vi "Routing Channel Page.vi"(8 "error in (no error)":errorcluster, 11 "Node Ptr":T8 format="%.0x") -> (0 "error out":errorcluster)   [LabVIEW 2017, in "Routing and Faulting System Explorer.lvlib"]
uses:
  Routing and Faulting System Explorer.lvlib
  <vilib>/NI Veristand/Custom Device API/Custom Device Item Ref.ctl
  State-Value Row.ctl
  Connection Row.ctl
  State Control.ctl
  Shared/UI Common/Duplicate Button.ctl
  Shared/UI Common/Add Button.ctl
  Shared/UI Common/Remove Button.ctl
  Routing Channel Page Controls.ctl
  2402a215-ce2b-4427-ab28-3f6d8102afb6.vi
  Shared/UI Common/Set Control Value.vi
  <vilib>/NI VeriStand/Custom Device API/Custom Device API.lvlib
  Scripting/Routing and Faulting Scripting.lvlib
  Shared/UI Common/UI Common.lvlib
panel:
  in  "Configuration Tab":T1(tab)
  in  "show module":bool
  in  "Connections":T2[](array[typedef])
  in  "State Value":string
  in  "State Description":string
  in  "Add Connection":T3
  in  "State Name":T4
  in  "Duplicate State":T5
  in  "Remove State":T6
  in  "Add State":T3
  out "States":T7[](array[typedef])
  in  "Initial State":string(combo)
  in  "Routing Channel Name":string
  in  "SHDocVw.IWebBrowser":refnum<k7>(container)
  in  "Description":string
  # "Source"
  # "Destination"
  # "State Name"
  # "State Value"
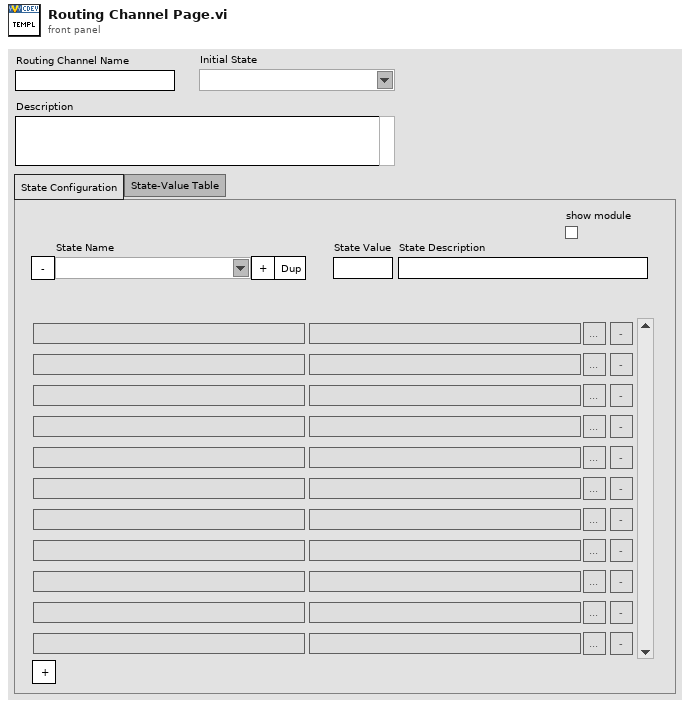
[diagram p1: front panel]
types:
  T1 = enum32{"State Configuration", "State-Value Table"}
  T2 = typedef "Routing and Faulting System Explorer.lvlib/Connection Row.ctl" = cluster{"Source":string, "Destination":string, "Edit":bool, "Remove":bool}
  T3 = typedef "UI Common.lvlib/Add Button.ctl" = bool
  T4 = typedef "Routing and Faulting System Explorer.lvlib/State Control.ctl" = string
  T5 = typedef "UI Common.lvlib/Duplicate Button.ctl" = bool
  T6 = typedef "UI Common.lvlib/Remove Button.ctl" = bool
  T7 = typedef "Routing and Faulting System Explorer.lvlib/State-Value Row.ctl" = cluster{"State":string, "State Value":string}
  T8 = typedef "Custom Device API.lvlib/Custom Device Item Ref.ctl" = u64
  T9 = typedef "Routing and Faulting System Explorer.lvlib/Routing Channel Page Controls.ctl" = cluster{"Description":refnum<vi>, "Routing Channel Name":refnum<vi>, "Initial State":refnum<vi>, "Configuration Tab":refnum<vi>, "States":refnum<vi>, "State Value":refnum<vi>, "State Name":refnum<vi>, "State Description":refnum<vi>, "Connections":refnum<vi>}
  T10 = typedef "Routing and Faulting System Explorer.lvlib/Channel Editor State.ctl" = cluster{"Controller":string, "Possible Connections":cluster{"Module":string, "Possible Connections":T11[]}[], "Alias Mappings UI":T12[], "Mappings by Module UI":T13[]}
  T11 = typedef "Routing and Faulting Hardware API.lvlib/Possible Connections for Endpoint.ctl" = cluster{"Source":string, "Destinations":string[]}
  T12 = typedef "Routing and Faulting Shared.lvlib/Alias Mapping.ctl" = cluster{"Endpoint":string, "Alias":string}
  T13 = typedef "Routing and Faulting System Explorer.lvlib/Alias Map by Module.ctl" = cluster{"Module":string, "Alias Map":cluster{"Aliases":string[], "Endpoints":string[]}}
  T14 = typedef "Custom Device API.lvlib/Custom Device Commands.ctl" = enum16{"Default", "Item renamed", "Shutdown", "Dynamic button pressed"}
  T15 = typedef "Routing and Faulting Shared.lvlib/Connection.ctl" = cluster{"Module":string, "Source":string, "Destination":string}
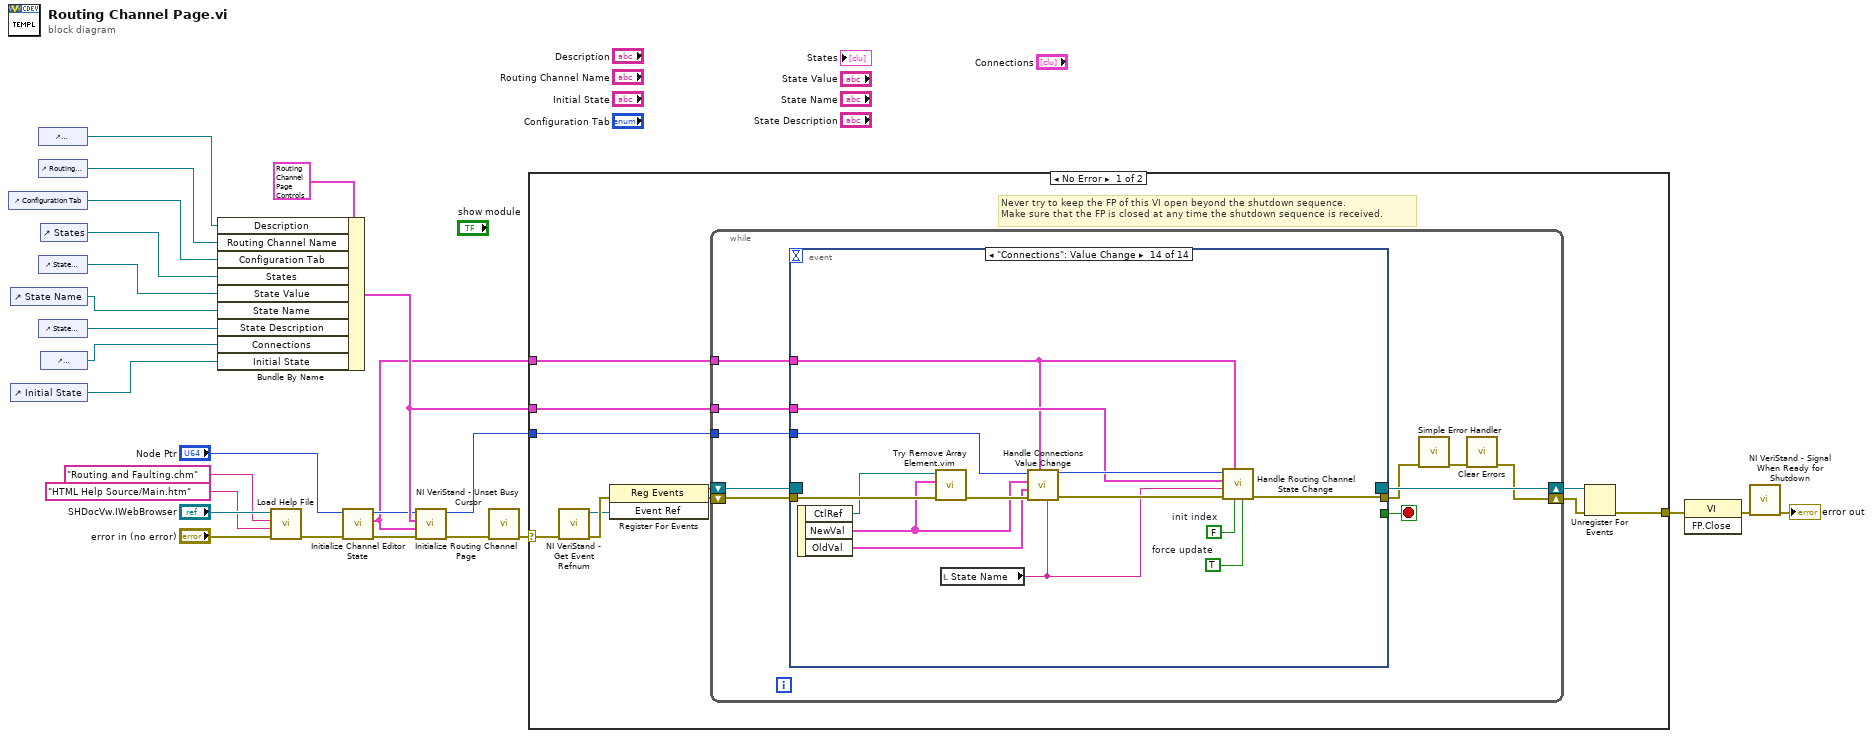
[diagram p0: block diagram]
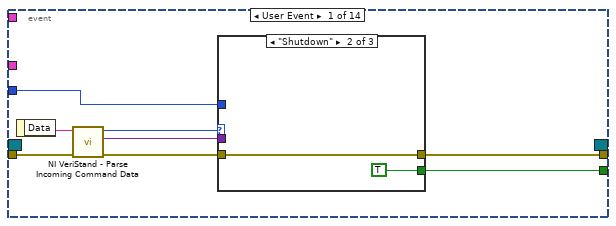
[diagram p2: hidden frame]
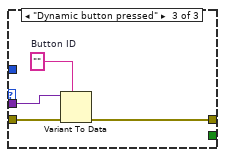
[diagram p4: hidden frame]
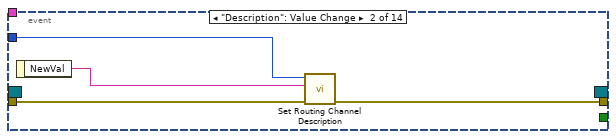
[diagram p5: hidden frame]
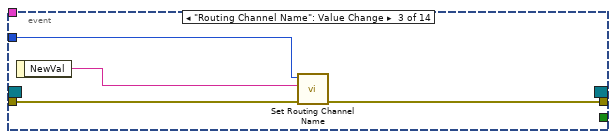
[diagram p6: hidden frame]
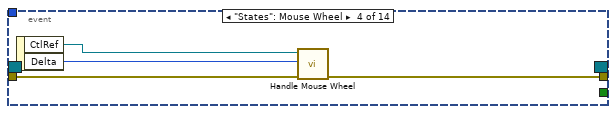
[diagram p7: hidden frame]
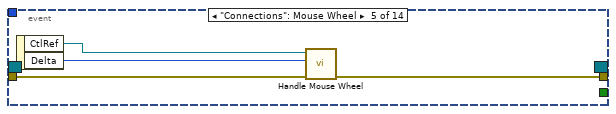
[diagram p8: hidden frame]
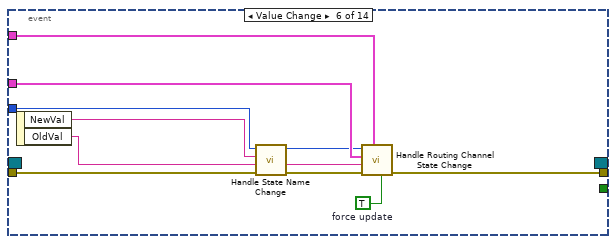
[diagram p9: hidden frame]
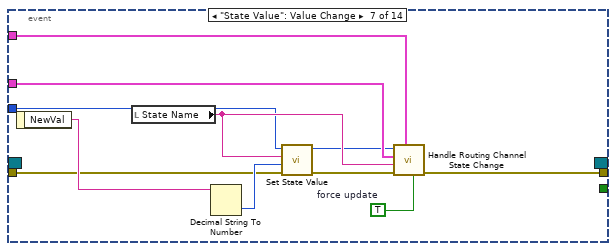
[diagram p10: hidden frame]
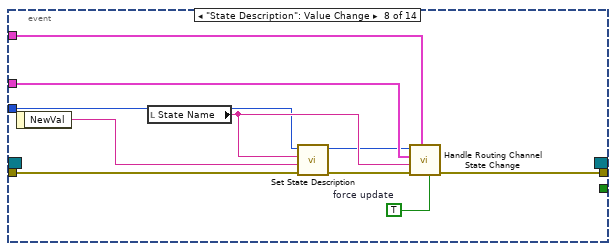
[diagram p11: hidden frame]
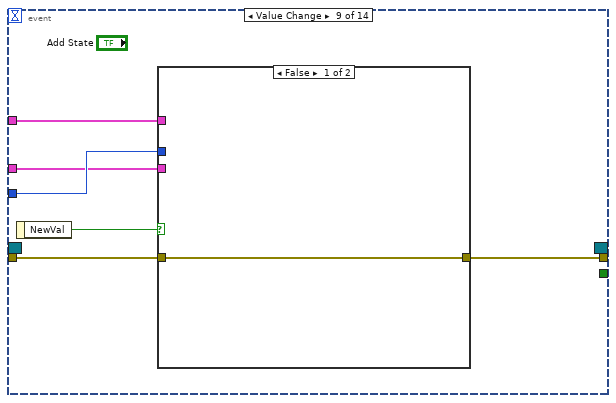
[diagram p12: hidden frame]
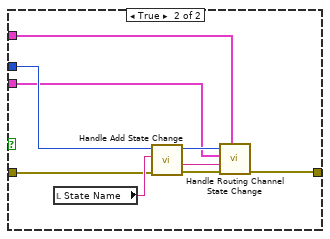
[diagram p13: hidden frame]
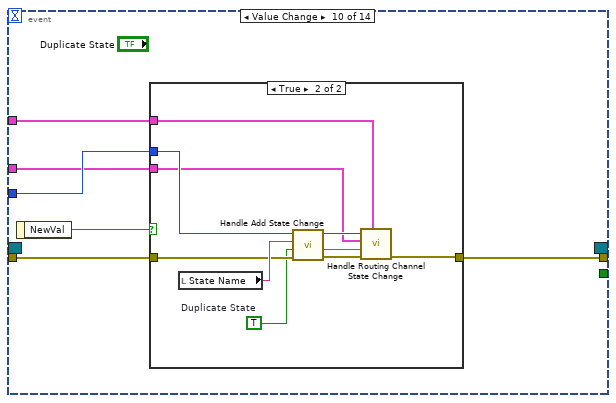
[diagram p14: hidden frame]
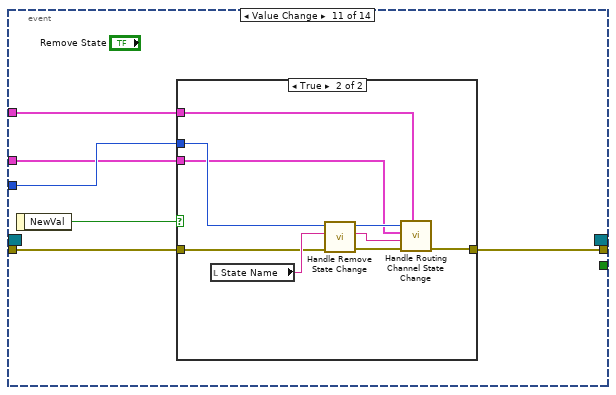
[diagram p16: hidden frame]
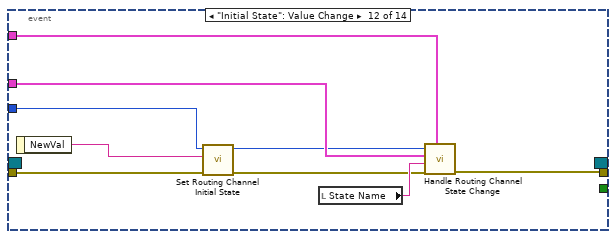
[diagram p18: hidden frame]
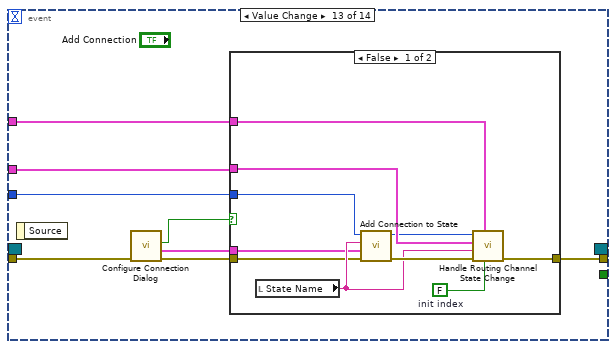
[diagram p19: hidden frame]
diagram:
  n1 = control-ref of="Configuration Tab"() -> (w21:refnum<vi>)
  n2 = control-ref of="State Name"() -> (w12:refnum<vi>)
  n3 = control-ref of="Initial State"() -> (w8:refnum<vi>)
  n4 = control-ref of="Description"() -> (w22:refnum<vi>)
  n5 = control-ref of="Routing Channel Name"() -> (w6:refnum<vi>)
  n6 = control-ref of="State Value"() -> (w19:refnum<vi>)
  n7 = control-ref of="State Description"() -> (w7:refnum<vi>)
  n8 = control-ref of="States"() -> (w20:refnum<vi>)
  n9 = control-ref of="Connections"() -> (w13:refnum<vi>)
  n10 = Bundle By Name(cluster=T9 {"Description"=refnum, "Routing Channel Name"=refnum, "Initial State"=refnum, "Configuration Tab"=refnum, "States"=refnum, "State Value"=refnum, "State Name"=refnum, "State Description"=refnum, "Connections"=refnum} ("Routing Channel Page Controls"), "Description"=w22, "Routing Channel Name"=w6, "Configuration Tab"=w21, "States"=w20, "State Value"=w19, "State Name"=w12, "State Description"=w7, "Connections"=w13, "Initial State"=w8) -> (w9:T9)
  n11 = call "Load Help File.vi"("error in (no error)"="error in (no error)", "HTML File to Load"="HTML Help Source/Main.htm" ("HTML File"), "Main CHM File"="Routing and Faulting.chm" ("CD_CHM_FileName"), "Browser"="SHDocVw.IWebBrowser") -> ("error out"=w4:errorcluster)  [unwired: 7 in]
  n12 = call "Initialize Channel Editor State.vi"("error in (no error)"=w4, "Routing Channel Ref in"="Node Ptr") -> ("error out"=w2:errorcluster, "Channel Editor State"=w1:T10, "Routing Channel Ref out"=w3:T8)  [unwired: 7 in]
  n13 = call "Initialize Routing Channel Page.vi"("error in (no error)"=w2, "Channel Editor State"=w1, "Routing Channel Page Controls"=w9, "Routing Channel Ref in"=w3) -> ("error out"=w10:errorcluster, "Routing Channel Ref out"=w11:T8)  [unwired: 6 in]
  n14 = call <vilib>:"NI VeriStand - Unset Busy Cursor.vi"("error in (no error)"=w10) -> ("error out"=w23:errorcluster)  [unwired: 10 out]
  n15 = case shown="No Error" w23 {
    selector: w23 -> [w29 w204]
    tunnel: [w34 w202] -> w26
    tunnel: w11 -> [w30 _]
    tunnel: w9 -> [w28 _]
    tunnel: w1 -> [w27 _]
    frame No Error {
      # "Never try to keep the FP of this VI open beyond the shutdown sequence.\nMake sure that the FP is closed at any time the shutdown sequence is received."
      n16 = call <vilib>:"NI VeriStand - Get Event Refnum.vi"("error in (no error)"=w29) -> ("error out"=w37:errorcluster, "Event Ref"=w33:refnum<user-event>)  [unwired: 9 out]
      n17 = register-events(error in=w37, w33) -> (reference out=w31:refnum<event-registration>, error out=w32:errorcluster)  [unwired: 1 in]
      n18 = while {
        tunnel: w30 -> [w43]
        shift-right: [w40] -> w35
        shift-left: w32 -> [w46]
        shift-right: [w47] -> w36
        shift-left: w31 -> [w45]
        tunnel: w28 -> [w39]
        tunnel: w27 -> [w38]
        stop <- w44 stop-if-true
        n19 = event shown="[13] \"Connections\": Value Change" {
          selector: w45 -> [_ _ _ _ _ _ _ _ _ _ _ _ _ _]
          dyn-events: [_ _ _ _ _ _ _ _ _ _ _ _ _ _] -> w47
          timeout: _ -> [_ _ _ _ _ _ _ _ _ _ _ _ _ _]
          tunnel: w46 -> [w55 w65 w68 w73 w77 w87 w96 w108 w115 w131 w147 w167 w174 w201]
          tunnel: [w51 _ _ _ _ _ _ _ _ _ _ _ _ _] -> w44
          tunnel: [w50 w64 w69 w74 w78 w89 w100 w110 w114 w130 w146 w166 w172 w194] -> w42
          tunnel: w43 -> [w49 w66 w70 _ _ w84 w93 w105 w116 w132 w149 w163 w176 w199]
          tunnel: w39 -> [_ _ _ _ _ w88 w99 w109 w112 w128 w148 w168 w173 w192]
          tunnel: w38 -> [_ _ _ _ _ w79 w90 w101 w111 w127 w144 w160 w169 w188]
          event User Event {
            n20 = event-data() -> ("Data"=w54:string)  [unwired: 1 out]
            n21 = call <vilib>:"NI VeriStand - Parse Incoming Command Data.vi"("error in (no error)"=w55, "Incoming data"=w54) -> ("error out"=w53:errorcluster, "Outgoing data"=w48:variant, "Action"=w52:T14)  [unwired: 7 out]
            n22 = case shown="\"Shutdown\"" w52 {
              tunnel: w53 -> [w56 w57 w62]
              tunnel: [_ TRUE _] -> w51
              tunnel: [w56 w57 w59] -> w50
              tunnel: w49 -> [_ _ _]
              tunnel: w48 -> [_ _ w61]
              frame "Default", Default {
              }
              frame "Shutdown" {
              }
              frame "Dynamic button pressed" {
                w60 = ""  # Button ID
                n23 = Variant To Data(error in=w62, type=w60, Variant=w61) -> (error out=w59:errorcluster)  [unwired: 1 out]
              }
            }
          }
          event "Description": Value Change {
            n24 = event-data() -> ("NewVal"=w63:string)  [unwired: 1 out]
            n25 = call "Set Routing Channel Description.vi"("error in (no error)"=w65, "Description"=w63, "Channel Ref in"=w66) -> ("error out"=w64:errorcluster)  [unwired: 7 in, 1 out]
          }
          event "Routing Channel Name": Value Change {
            n26 = event-data() -> ("NewVal"=w67:string)  [unwired: 1 out]
            n27 = call "Set Routing Channel Name.vi"("error in (no error)"=w68, "Channel Name"=w67, "Channel Ref in"=w70) -> ("error out"=w69:errorcluster)  [unwired: 7 in, 1 out]
          }
          event "States": Mouse Wheel {
            n28 = event-data() -> ("CtlRef"=w72:refnum<vi>, "Delta"=w71:i32)  [unwired: 1 out]
            n29 = call "Handle Mouse Wheel.vi"("error in (no error)"=w73, "delta"=w71, "Array Refnum"=w72) -> ("error out"=w74:errorcluster)  [unwired: 7 in, 1 out]
          }
          event "Connections": Mouse Wheel {
            n30 = event-data() -> ("CtlRef"=w75:refnum<vi>, "Delta"=w76:i32)  [unwired: 1 out]
            n31 = call "Handle Mouse Wheel.vi"("error in (no error)"=w77, "delta"=w76, "Array Refnum"=w75) -> ("error out"=w78:errorcluster)  [unwired: 7 in, 1 out]
          }
          event Value Change {
            w80 = TRUE  # force update
            n32 = event-data() -> ("NewVal"=w86:T4, "OldVal"=w85:T4)  [unwired: 1 out]
            n33 = call "Handle State Name Change.vi"("error in (no error)"=w87, "Old State Name"=w85, "New State Name"=w86, "Routing Channel Ref in"=w84) -> ("error out"=w83:errorcluster, "State to Display"=w81:string, "Routing Channel Ref out"=w82:T8)  [unwired: 5 in]
            n34 = call "Handle Routing Channel State Change.vi"("force update"=w80, "Channel Editor State"=w79, "error in (no error)"=w83, "State"=w81, "Routing Channel Page Controls"=w88, "Routing Channel Ref in"=w82) -> ("error out"=w89:errorcluster)  [unwired: 4 in, 1 out]
          }
          event "State Value": Value Change {
            w91 = TRUE  # force update
            n35 = event-data() -> ("NewVal"=w97:string)  [unwired: 1 out]
            n36 = local read "State Name"() -> (w94:T4)
            n37 = Decimal String To Number(string=w97) -> (number=w98:i32)  [unwired: 2 in, 1 out]
            n38 = call "Set State Value.vi"("error in (no error)"=w96, "New Value"=w98, "State"=w94, "Channel Ref in"=w93) -> ("error out"=w95:errorcluster, "Channel Ref out"=w92:T8)  [unwired: 6 in]
            n39 = call "Handle Routing Channel State Change.vi"("force update"=w91, "Channel Editor State"=w90, "error in (no error)"=w95, "State"=w94, "Routing Channel Page Controls"=w99, "Routing Channel Ref in"=w92) -> ("error out"=w100:errorcluster)  [unwired: 4 in, 1 out]
          }
          event "State Description": Value Change {
            w103 = TRUE  # force update
            n40 = event-data() -> ("NewVal"=w102:string)  [unwired: 1 out]
            n41 = local read "State Name"() -> (w106:T4)
            n42 = call "Set State Description.vi"("error in (no error)"=w108, "Description"=w102, "State"=w106, "Channel Ref in"=w105) -> ("error out"=w107:errorcluster, "Channel Ref out"=w104:T8)  [unwired: 6 in]
            n43 = call "Handle Routing Channel State Change.vi"("force update"=w103, "Channel Editor State"=w101, "error in (no error)"=w107, "State"=w106, "Routing Channel Page Controls"=w109, "Routing Channel Ref in"=w104) -> ("error out"=w110:errorcluster)  [unwired: 4 in, 1 out]
          }
          event Value Change {
            n44 = event-data() -> ("NewVal"=w113:T3)  [unwired: 1 out]
            n45 = case shown="False" w113 {
              tunnel: w116 -> [_ w126]
              tunnel: w112 -> [_ w122]
              tunnel: w115 -> [w117 w120]
              tunnel: [w117 w121] -> w114
              tunnel: w111 -> [_ w118]
              frame False {
              }
              frame True {
                n46 = local read "State Name"() -> (w125:T4)
                n47 = call "Handle Add State Change.vi"("error in (no error)"=w120, "State"=w125, "Routing Channel Ref in"=w126) -> ("error out"=w123:errorcluster, "New State Added"=w119:string, "Routing Channel Ref out"=w124:T8)  [unwired: 6 in]
                n48 = call "Handle Routing Channel State Change.vi"("Channel Editor State"=w118, "error in (no error)"=w123, "State"=w119, "Routing Channel Page Controls"=w122, "Routing Channel Ref in"=w124) -> ("error out"=w121:errorcluster)  [unwired: 5 in, 1 out]
              }
            }
          }
          event Value Change {
            n49 = event-data() -> ("NewVal"=w129:T5)  [unwired: 1 out]
            n50 = case shown="True" w129 {
              tunnel: w132 -> [_ w143]
              tunnel: w128 -> [_ w139]
              tunnel: w131 -> [w133 w137]
              tunnel: [w133 w138] -> w130
              tunnel: w127 -> [_ w134]
              frame False {
              }
              frame True {
                w135 = TRUE  # Duplicate State
                n51 = local read "State Name"() -> (w142:T4)
                n52 = call "Handle Add State Change.vi"("error in (no error)"=w137, "Duplicate State"=w135, "State"=w142, "Routing Channel Ref in"=w143) -> ("error out"=w140:errorcluster, "New State Added"=w136:string, "Routing Channel Ref out"=w141:T8)  [unwired: 5 in]
                n53 = call "Handle Routing Channel State Change.vi"("Channel Editor State"=w134, "error in (no error)"=w140, "State"=w136, "Routing Channel Page Controls"=w139, "Routing Channel Ref in"=w141) -> ("error out"=w138:errorcluster)  [unwired: 5 in, 1 out]
              }
            }
          }
          event Value Change {
            n54 = event-data() -> ("NewVal"=w145:T6)  [unwired: 1 out]
            n55 = case shown="True" w145 {
              tunnel: w149 -> [_ w159]
              tunnel: w148 -> [_ w155]
              tunnel: w147 -> [w150 w153]
              tunnel: [w150 w154] -> w146
              tunnel: w144 -> [_ w151]
              frame False {
              }
              frame True {
                n56 = local read "State Name"() -> (w158:T4)
                n57 = call "Handle Remove State Change.vi"("error in (no error)"=w153, "State"=w158, "Routing Channel Ref in"=w159) -> ("error out"=w156:errorcluster, "State to Display"=w152:string, "Routing Channel Ref out"=w157:T8)  [unwired: 6 in]
                n58 = call "Handle Routing Channel State Change.vi"("Channel Editor State"=w151, "error in (no error)"=w156, "State"=w152, "Routing Channel Page Controls"=w155, "Routing Channel Ref in"=w157) -> ("error out"=w154:errorcluster)  [unwired: 5 in, 1 out]
              }
            }
          }
          event "Initial State": Value Change {
            n59 = event-data() -> ("NewVal"=w161:string)  [unwired: 1 out]
            n60 = call "Set Routing Channel Initial State.vi"("error in (no error)"=w167, "State"=w161, "Channel Ref in"=w163) -> ("error out"=w164:errorcluster, "Channel Ref out"=w162:T8)  [unwired: 7 in]
            n61 = local read "State Name"() -> (w165:T4)
            n62 = call "Handle Routing Channel State Change.vi"("Channel Editor State"=w160, "error in (no error)"=w164, "State"=w165, "Routing Channel Page Controls"=w168, "Routing Channel Ref in"=w162) -> ("error out"=w166:errorcluster)  [unwired: 5 in, 1 out]
          }
          event Value Change {
            n63 = event-data() -> ()  [unwired: 2 out]
            n64 = call "Configure Connection Dialog.vi"("error in (no error)"=w174) -> ("error out"=w175:errorcluster, "Connection (R,S,D)"=w170:T15, "Canceled?"=w171:bool)  [unwired: 8 in]
            n65 = case shown="False" w171 {
              tunnel: w176 -> [w183 _]
              tunnel: w170 -> [w179 _]
              tunnel: w175 -> [w180 w187]
              tunnel: w173 -> [w185 _]
              tunnel: [w182 w187] -> w172
              tunnel: w169 -> [w177 _]
              frame False {
                w178 = FALSE  # init index
                n66 = local read "State Name"() -> (w181:T4)
                n67 = call "Add Connection to State.vi"("error in (no error)"=w180, "Connection"=w179, "State"=w181, "Channel Ref in"=w183) -> ("error out"=w186:errorcluster, "Channel Ref out"=w184:T8)  [unwired: 6 in]
                n68 = call "Handle Routing Channel State Change.vi"("init index"=w178, "Channel Editor State"=w177, "error in (no error)"=w186, "State"=w181, "Routing Channel Page Controls"=w185, "Routing Channel Ref in"=w184) -> ("error out"=w182:errorcluster)  [unwired: 4 in, 1 out]
              }
              frame True {
              }
            }
          }
          event "Connections": Value Change {
            w189 = TRUE  # force update
            w196 = FALSE  # init index
            n69 = event-data() -> ("CtlRef"=w191:refnum<vi>, "NewVal"=w198:T2[], "OldVal"=w197:T2[])  [unwired: 1 out]
            n70 = call "Try Remove Array Element.vim"("error in (no error)"=w201, "Array"=w198, "Ctl Refnum"=w191) -> ("error out"=w200:errorcluster)  [unwired: 6 in, 2 out]
            n71 = local read "State Name"() -> (w190:T4)
            n72 = call "Handle Connections Value Change.vi"("State"=w190, "Channel Editor State"=w188, "error in (no error)"=w200, "OldVal"=w197, "NewVal"=w198, "Routing Channel Ref in"=w199) -> ("error out"=w195:errorcluster, "Routing Channel Ref out"=w193:T8)  [unwired: 4 in]
            n73 = call "Handle Routing Channel State Change.vi"("force update"=w189, "init index"=w196, "Channel Editor State"=w188, "error in (no error)"=w195, "State"=w190, "Routing Channel Page Controls"=w192, "Routing Channel Ref in"=w193) -> ("error out"=w194:errorcluster)  [unwired: 3 in, 1 out]
          }
        }
        n74 = call <vilib>:"Simple Error Handler.vi"("error in (no error)"=w42) -> ("error out"=w41:errorcluster)  [unwired: 1 in, 7 out]
        n75 = call <vilib>:"Clear Errors.vi"("error in (no error)"=w41) -> ("error out"=w40:errorcluster)  [unwired: 1 in, 5 out]
      }
      n76 = Unregister For Events(event registration refnum=w36, error in=w35) -> (error out=w34:errorcluster)
    }
    frame Error {
      n77 = call <vilib>:"Simple Error Handler.vi"("error in (no error)"=w204) -> ("error out"=w203:errorcluster)  [unwired: 1 in, 7 out]
      n78 = call <vilib>:"Clear Errors.vi"("error in (no error)"=w203) -> ("error out"=w202:errorcluster)  [unwired: 1 in, 5 out]
    }
  }
  n79 = invoke class="VI" method="FP.Close"(error in=w26) -> (error out=w25:errorcluster)  [unwired: 2 in, 2 out]
  n80 = call <vilib>:"NI VeriStand - Signal When Ready for Shutdown.vi"("error in (no error)"=w25) -> ("error out"=→"error out":errorcluster)  [unwired: 10 out]
